vi "Dashboard Main.vi"() -> ()   [LabVIEW 2015]
uses:
  Common Code/Auton Command Cluster.ctl
  Common Code/Auton File Lists.ctl
  Vision/Camera Types.ctl
  Common Code/Goal Vision Packet.ctl
  <vilib>/Rock Robotics/WPI/Camera/WPI_CameraSettings Read MJPG.ctl
  <vilib>/Rock Robotics/WPI/Camera/WPI_CameraImageSize.ctl
  Common Code/Encoder Values Super Cluster.ctl
  Common Code/Encoder Values.ctl
  Common Code/Power and Diagnostic Data.ctl
  Common Code/Utilities/PDP Data.ctl
  Common Code/Utilities/PCM Data.ctl
  Common Code/IMU Data.ctl
  navX.Library.v2/navX Library v2/TypeDefs/Flags/Z900_navX_Flags_CalibrationStatusTypeDef.ctl
  navX.Library.v2/navX Library v2/TypeDefs/Flags/Z900_navX_Flags_OpStatusTypeDef.ctl
  Common Code/Intake Status Cluster.ctl
  Common Code/Intake Mode.ctl
  Common Code/Intake States.ctl
  Common Code/Climb Status Cluster.ctl
  Common Code/Climb Mode.ctl
  Common Code/Climb Presets.ctl
  Common Code/Major Loop Times.ctl
  Common Code/Drivetrain Settings.ctl
  Common Code/Intake Presets.ctl
  Common Code/Drivetrain Output Range.ctl
  Common Code/Ultrasonic Data.ctl
  Common Code/Autonomous Presets.ctl
  Common Code/Robot Name.ctl
  Common Code/Encoder Control.ctl
  Common Code/Drivetrain Status Cluster.ctl
  Common Code/Drivetrain Modes.ctl
  Common Code/Dist Drive Status.ctl
  Common Code/Auto Shift Cluster.ctl
  Common Code/Catapult/Catapult Presets.ctl
  Common Code/Dashboard Communication/Dashboard Control Data.ctl
  Common Code/Dashboard Drivetrain Command.ctl
  Common Code/Drivetrain Vision.ctl
  Common Code/Ball Tracking Command Cluster.ctl
  Common Code/Ball Vision Packet.ctl
  Common Code/Tracking Mode.ctl
  Common Code/IntakeEcoderControl.ctl
  Common Code/Enabled Systems.ctl
  Common Code/Dashboard Communication/Dashboard Display Data.ctl
  <vilib>/Rock Robotics/WPI/Dashboard/WPI_DashboardLogging Global.vi
  <vilib>/Utility/inputDevices.llb/keyboardAcquire.vi
  navX.Library.v2/navX Library v2/navX Library v2.lvlib
panel:
  in  "Robot":T1
  in  "Logging Filename":path=path ""
  in  "stop":bool
  out "DumbDashMessage":string="137 values loaded OK"
  in  "Save":bool
  in  "Load":bool
  in  "TCP":refnum<k5>
  in  "Rec Mode":enum32{"Stop", "Record", "Playback"}(radio)
  out "Image Message":string="Timeout in Camera Communications"
  in  "Dashboard Tab":T2(tab)
  out "Pressure":dbl
  out "Goal Active? 2":bool
  out "Drivetrain Mode":bool
  out "Intake State":bool
  out "Mode":T3(ring)=enum."Disconnected"
  out "Gyro":dbl(knob) scale=0.0..360.0 scale format="%#.7g"
  out "Climb Mode":bool
  out "Intake Mode":bool
  out "Camera IP":string="0.0.0.0"
  out "Robot IP":string="0.0.0.0"
  out "Front Camera Display":T4(plugin-control)
  in  "Camera Mode":u16(ring)=3 items=["Camera Off", "USB Camera SW", "USB Camera HW", "IP Camera"]
  out "FPS":dbl
  out "Bandwidth (Mbps)":dbl
  out "navX Calibration Status":T5 items=["IMU_CAL_STATE_MASK"=3, "IMU_CAL_STATE_INPROGRESS"=0, "IMU_CAL_STATE_ACCUMULATE"=1, "IMU_CAL_STATE_COMPLETE"=2]
  out "Front Camera Display 2":T4(plugin-control)
  out "Line Number":i32
  in  "Auton Presets":T6
  out "Auton Command Cluster":T7
  out "Auton File Lists":T8
  in  "Auto-Shift":T9
  in  "Encoder Settings":T10
  in  "Drivetrain Settings":T11={"Gyro Tolerance"=6.0, "Throttle Ramp (ms)"=250.0, "Kv"=0.0, "Ka"=0.0, "Feed Forward P"=1.0, "Feed Forward D"=0.0, "Goal Vision PID gains"={"proportional gain (Kc)"=0.8, "integral time (Ti, min)"=0.05, "derivative time (Td, min)"=0.003}, "Goal Detection Window"=12.0, "Creep Rate"=0.0, "Vision Throttle Threshold"=0.0, "Min Turn Output"=0.0, "Left Batter Angle"=0.0, "Right Batter Angle"=0.0} {"Goal Vision PID gains"."derivative time (Td, min)" format="%.5f"; "Goal Vision PID gains"."integral time (Ti, min)" format="%.3f"; "Goal Vision PID gains"."proportional gain (Kc)" format="%.3f"}
  in  "Goal Output Range":cluster{"output high":dbl, "output low":dbl}={"output high"=0.8, "output low"=-0.8}
  out "Encoder Values":T12
  in  "Steer PID output":cluster{"output high":dbl, "output low":dbl}
  in  "Steer PID gains":T14
  out "Drivetrain Status Cluster":T15={"Modes"=enum."Manual", "Y (Throttle)"=0.0, "X (Steer)"=0.0, "Gyro In Range?"=FALSE, "Distance Drive Finished?"=FALSE, "Stop Eject Lockout"=FALSE, "Dist Drive Status"={"Y In Range"=FALSE, "X In Range"=FALSE, "Gyro In Range"=FALSE, "Y Dist"=0.0, "X Dist"=0.0, "Gyro"=0.0}, "Y Target"=0.0, "Heading Target"=0.0, "Vision Target Aligned?"=FALSE}
  in  "Catapult Setpoints":T18
  in  "Intake Presets":T19={"Intake Speed"=0.8, "Outake Speed"=-0.8, "Low Height"=5.0, "Half Height"=55.0, "High Idle Height"=90.0, "Angle Speed"=0.0, "Angle Tolerance"=5.0, "Encoder Scale"=0.001478, "Load Height"=4.0, "Output Range"={"output high"=0.4, "output low"=-0.4}, "Rotation Power Max/Min"=0.5, "MaxCurrent"=40.0, "Intake Trip Time"=500.0, "Idle Height"=27.0, "Max Height"=90.0, "Reset Encoders?"=FALSE, "PID gains"={"proportional gain (Kc)"=1.0, "integral time (Ti, min)"=0.0, "derivative time (Td, min)"=0.003}, "Intake Stop Delay"=0, "Settle Time"=0.0, "Settle Wait Time"=0.0, "Pull Up Delay"=0.0} {"Pull Up Delay" format="%#_7g"; "Settle Wait Time" format="%#_7g"; "Settle Time" format="%#_7g"; "Intake Stop Delay" format="%#_7g"; "Max Height" format="%#_7g"; "Idle Height" format="%#_7g"; "Intake Trip Time" format="%#_7g"; "MaxCurrent" format="%#_7g"; "Rotation Power Max/Min" format="%#_7g"; "Load Height" format="%#_7g"; "Encoder Scale" format="%#_7g"; "Angle Tolerance" format="%#_7g"; "Angle Speed" format="%#_7g"; "High Idle Height" format="%#_7g"; "Half Height" format="%#_7g"; "Low Height" format="%#_7g"; "Outake Speed" format="%#_7g"; "Intake Speed" format="%#_7g"}
  out "Intake Status Cluster":T21
  in  "Climb Presets":T24={"Pull Power"=0.0, "Extend Power"=1.0}
  out "Climb Status Cluster":T25
  in  "Pressure B":dbl
  in  "Pressure M":dbl=22.0
  out "Pressure Sensor Voltage":dbl
  out "IMU Data":T27 {"OP Status" items=["INITIALIZING", "SELFTEST_IN_PROGRESS", "ERROR", "IMU_AUTOCAL_IN_PROGRESS", "NORMAL"]; "Calibration Status" items=["IMU_CAL_STATE_MASK"=3, "IMU_CAL_STATE_INPROGRESS"=0, "IMU_CAL_STATE_ACCUMULATE"=1, "IMU_CAL_STATE_COMPLETE"=2]}
  out "Gyro 2":dbl(knob) scale=0.0..360.0 scale format="%#.7g"
  out "Ultrasonic Data":T29
  out "Ball Cam Active?":bool
  out "Camera Display 2":T4(plugin-control)
  in  "Aspect Fudge Factor":dbl=1.0
  in  "Score Threshold 2":dbl=75.0 format="%#_13g"
  out "Goal Display":T4(plugin-control)
  out "Found Targets":T30(array[cluster]) {"Normalized Rect"."Numeric 5" format="%#_2g"; "Normalized Rect"."Numeric 3" format="%#_2g"; "Normalized Rect"."Numeric 2" format="%#_2g"; "Normalized Rect"."Numeric" format="%#_2g"}
  in  "Camera Type":T31=enum."1013"
  out "Goal Vision Packet":T32
  in  "Goal Camera Settings":T33={"fps"=30, "compression"=30, "Image Size"=enum."320x240"}
  in  "File number":i32
  in  "Use Goal File?":bool
  in  "Color Components":T35={"Hue"={34.0, 185.0}, "Sat"={0.0, 181.0}, "Val"={142.0, 255.0}} {"Val" scale=0.0..255.0; "Sat" scale=0.0..255.0; "Hue" scale=0.0..255.0 scale format="%#_3g"}
  out "Goal Active?":bool
  in  "Camera Mode 2":u16(ring) items=["Camera Off", "USB Camera SW", "USB Camera HW", "IP Camera"]
  out "FPS 2":dbl
  out "Bandwidth (Mbps) 2":dbl
  in  "Ball Camera Settings":T33={"fps"=30, "compression"=30, "Image Size"=enum."320x240"}
  out "Front Camera Display 3":T4(plugin-control)
  in  "Vision Timeout":dbl
  out "Power and Diagnostic Data":T36
  out "Control Info":T39
  out "Status Info":T40
  out "DS TCP":T41={"Error Strings"="", "Disable Counts"={0, 0}, "Rail Faults"={0, 0, 0}, "Robot IP"="0.0.0.0", "DB Mode"=4, "Event Info"={"Name"="", "Type"=0, "Number"=0, "Replay"=0}, "Camera Addr"="0.0.0.0"}
  out "Robot Metrics":T42
  out "Loop Times":T43
  # "USB Cam"
  # "Axis Cam"
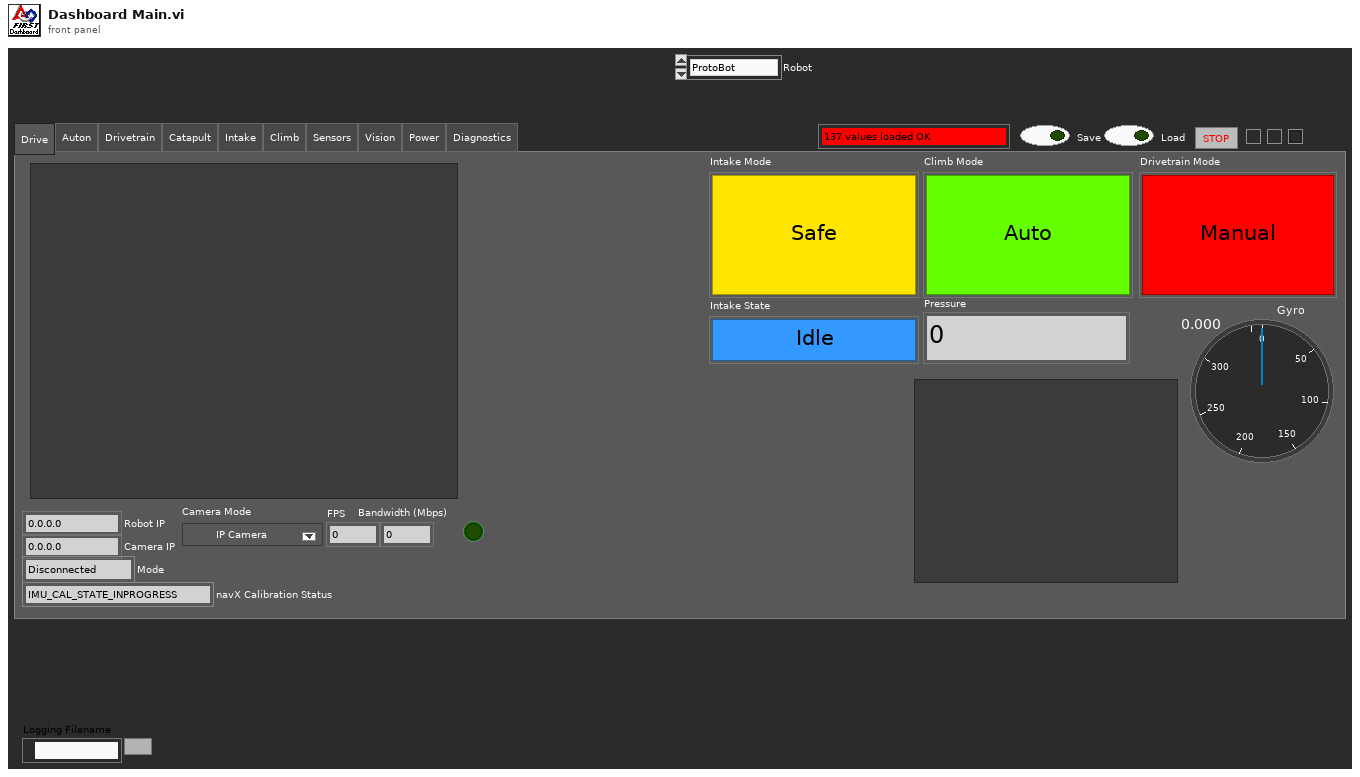
[diagram p1: front panel]
types:
  T1 = typedef "Robot Name.ctl" = enum16{"ProtoBot", "Main Robot", "Practice Robot"}
  T2 = enum32{"Drive", "Auton", "Drivetrain", "Catapult", "Intake", "Climb", "Sensors", "Vision", "Power", "Diagnostics"}
  T3 = enum8{"Tele-Op Disabled", "Tele-Op Enabled", "Auto Disabled", "Auto Enabled", "Test Disabled", "Test Enabled", "Disconnected", "No Code", "E-Stop"}
  T4 = typedef "IMAQ Image.ctl" = refnum<image>
  T5 = typedef "navX Library v2.lvlib/Z900_navX_Flags_CalibrationStatusTypeDef.ctl" = u8
  T6 = typedef "Autonomous Presets.ctl" = cluster{"Pitch Limit":dbl, "Roll Limit":dbl, "Start Position":dbl, "Cross Position":dbl}
  T7 = typedef "Auton Command Cluster.ctl" = cluster{"Command ID":i32, "maxTime":dbl, "Y Distance":dbl, "Heading":dbl, "Throttle":dbl, "Async":dbl, "Velocity":dbl, "Acceleration":dbl, "To":dbl, "Condition":dbl, "Shot Type":dbl, "Left RPM":dbl, "Override RPM":i32, "Override Angle":i32, "Right RPM":dbl, "Angle":dbl, "Intake Mode":i32, "Intake Cmd":i32, "Intake O":i32, "Eject O":i32, "Angle O":i32, "Arm O":i32, "Intake Speed":dbl, "Eject Speed":dbl, "Arm Angle":dbl, "Arm Speed":dbl, "Intake?":i32, "Eject?":i32, "Left":dbl, "Right":dbl, "Pivot Speed":dbl, "Y Dist":dbl, "Position":dbl, "Desired Position":i32, "Shooter Mode":dbl, "Shooter Command":dbl, "Shoot?":dbl, "Shoot mode":dbl}
  T8 = typedef "Auton File Lists.ctl" = cluster{"Current Queue":string, "General Scripts":string, "Defense Scripts":string, "Movement Scripts":string}
  T9 = typedef "Auto Shift Cluster.ctl" = cluster{"Delay":dbl, "Speed Thresh":dbl, "Upshift Accel":dbl, "Upshift Throttle":dbl, "Upshift Throttle Accel":dbl, "Downshift Throttle":dbl, "Downshift Throttle Accel":dbl, "Pressure Threshold":dbl}
  T10 = typedef "Encoder Control.ctl" = cluster{"Right Tick Constant":dbl, "Left Tick Constant":dbl, "Reset?":bool, "Y Dist":cluster{"PID gains":cluster{"proportional gain (Kc)":dbl, "integral time (Ti, min)":dbl, "derivative time (Td, min)":dbl}}, "Y Stop Thresh":dbl, "Y Stop Speed":dbl}
  T11 = typedef "Drivetrain Settings.ctl" = cluster{"Gyro Tolerance":dbl, "Throttle Ramp (ms)":dbl, "Kv":dbl, "Ka":dbl, "Feed Forward P":dbl, "Feed Forward D":dbl, "Goal Vision PID gains":cluster{"proportional gain (Kc)":dbl, "integral time (Ti, min)":dbl, "derivative time (Td, min)":dbl}, "Goal Detection Window":dbl, "Creep Rate":dbl, "Vision Throttle Threshold":dbl, "Min Turn Output":dbl, "Left Batter Angle":dbl, "Right Batter Angle":dbl}
  T12 = typedef "Encoder Values Super Cluster.ctl" = cluster{"Left Encoder":T13, "Right Encoder":T13}
  T13 = typedef "Encoder Values.ctl" = cluster{"Distance":dbl, "Speed":dbl, "Ticks":dbl}
  T14 = cluster{"proportional gain (Kc)":dbl, "integral time (Ti, min)":dbl, "derivative time (Td, min)":dbl}
  T15 = typedef "Drivetrain Status Cluster.ctl" = cluster{"Modes":T16, "Y (Throttle)":dbl, "X (Steer)":dbl, "Gyro In Range?":bool, "Distance Drive Finished?":bool, "Stop Eject Lockout":bool, "Dist Drive Status":T17, "Y Target":dbl, "Heading Target":dbl, "Vision Target Aligned?":bool}
  T16 = typedef "Drivetrain Modes.ctl" = enum16{"Gyro Steer", "Climb", "Manual", "Goal Vision Targeting", "PID Distance Drive", "Hybrid"}
  T17 = typedef "Dist Drive Status.ctl" = cluster{"Y In Range":bool, "X In Range":bool, "Gyro In Range":bool, "Y Dist":dbl, "X Dist":dbl, "Gyro":dbl}
  T18 = typedef "Catapult Presets.ctl" = cluster{"Intake Danger Height":dbl, "Ball Security Delay ":dbl, "High PSI Minimum":dbl, "Shot Finish Delay":dbl, "Low PSI Minimum":dbl, "Idle Ball Security Wait ":dbl}
  T19 = typedef "Intake Presets.ctl" = cluster{"Intake Speed":dbl, "Outake Speed":dbl, "Low Height":dbl, "Half Height":dbl, "High Idle Height":dbl, "Angle Speed":dbl, "Angle Tolerance":dbl, "Encoder Scale":dbl, "Load Height":dbl, "Output Range":T20, "Rotation Power Max/Min":dbl, "MaxCurrent":dbl, "Intake Trip Time":dbl, "Idle Height":dbl, "Max Height":dbl, "Reset Encoders?":bool, "PID gains":cluster{"proportional gain (Kc)":dbl, "integral time (Ti, min)":dbl, "derivative time (Td, min)":dbl}, "Intake Stop Delay":u32, "Settle Time":dbl, "Settle Wait Time":dbl, "Pull Up Delay":dbl}
  T20 = typedef "Drivetrain Output Range.ctl" = cluster{"output high":dbl, "output low":dbl}
  T21 = typedef "Intake Status Cluster.ctl" = cluster{"Roller Power":dbl, "Angle Power":dbl, "Intake Mode":T22, "Intake States":T23, "Rollers Active?":bool, "Current Height":dbl, "Target Height":dbl, "Encoder Raw Position":dbl, "Forward Tripped?":bool, "Backward Tripped?":bool, "Override IR?":bool}
  T22 = typedef "Intake Mode.ctl" = enum16{"Safe", "Auto", "Manual"}
  T23 = typedef "Intake States.ctl" = enum16{"Idle", "Set roller speed", "Move to angle", "Go Hard or Go Home", "Ball Settle"}
  T24 = typedef "Climb Presets.ctl" = cluster{"Pull Power":dbl, "Extend Power":dbl}
  T25 = typedef "Climb Status Cluster.ctl" = cluster{"Pull Power":dbl, "Unpin Power":dbl, "PTO Engaged?":bool, "Climb Mode":T26}
  T26 = typedef "Climb Mode.ctl" = enum16{"Auto", "Semi-Auto", "Manual"}
  T27 = typedef "IMU Data.ctl" = cluster{"Pitch":sgl, "Roll":sgl, "Yaw":sgl, "Data Valid?":bool, "Temp":sgl, "MOVING":bool, "YAW_STABLE":bool, "Accel X":sgl, "Accel Y":sgl, "Accel Z":sgl, "Accel Magnitude":sgl, "Pitch Rate":sgl, "Roll Rate":sgl, "Yaw Rate":sgl, "NavX Opened?":bool, "Calibration Status":T5, "OP Status":T28}
  T28 = typedef "navX Library v2.lvlib/Z900_navX_Flags_OpStatusTypeDef.ctl" = u8
  T29 = typedef "Ultrasonic Data.ctl" = cluster{"Left Ultrasonic":dbl, "Right Ultrasonic":dbl}
  T30 = cluster{"Distance (ft)":dbl, "Center":cluster{dbl, dbl}, "Normalized Rect":cluster{"Numeric":dbl, "Numeric 2":dbl, "Numeric 3":dbl, "Numeric 5":dbl}}[]
  T31 = typedef "Camera Types.ctl" = enum16{"206", "1011", "1013", "MS HD3000 square", "MS HD3000 640x480"}
  T32 = typedef "Goal Vision Packet.ctl" = cluster{"Distance":dbl, "Center X":dbl, "Center Y":dbl, "Found Target?":bool, "Robot Center":dbl, "Angle":dbl}
  T33 = typedef "WPI_CameraSettings Read MJPG.ctl" = cluster{"fps":i32, "compression":i32, "Image Size":T34}
  T34 = typedef "WPI_CameraImageSize.ctl" = enum16{"640x480", "320x240", "160x120", "Custom"}
  T35 = cluster{"Hue":cluster{dbl, dbl}, "Sat":cluster{dbl, dbl}, "Val":cluster{dbl, dbl}}
  T36 = typedef "Power and Diagnostic Data.ctl" = cluster{"PDP Data":T37, "PCM Data":T38, "roboRIO input voltage (V)":dbl, "roboRIO input current (A)":dbl, "3.3V Rail Short":bool, "5 V Rail Short":bool, "6 V Rail Short":bool, "roboRIO Brownout":bool, "Outputs Enabled?":bool}
  T37 = typedef "PDP Data.ctl" = cluster{"Battery Voltage":sgl, "Temperature (degrees C)":sgl, "Internal Battery R (Ohms)":sgl, "Energy (J)":sgl, "Power (W)":sgl, "Total Current (A)":sgl, "Battery Voltage Fault":bool, "Temperature Fault":bool, "Hardware Fault":bool, "Currents":cluster{"[0]":sgl, "[1]":sgl, "[2]":sgl, "[3]":sgl, "[4]":sgl, "[5]":sgl, "[6]":sgl, "[7]":sgl, "[8]":sgl, "[9]":sgl, "[10]":sgl, "[11]":sgl, "[12]":sgl, "[13]":sgl, "[14]":sgl, "[15]":sgl}, "Current Faults":cluster{"[0]":bool, "[1]":bool, "[2]":bool, "[3]":bool, "[4]":bool, "[5]":bool, "[6]":bool, "[7]":bool, "[8]":bool, "[9]":bool, "[10]":bool, "[11]":bool, "[12]":bool, "[13]":bool, "[14]":bool, "[15]":bool}}
  T38 = typedef "PCM Data.ctl" = cluster{"Compressor Fault":bool, "Solenoid Fault":bool, "Compressor Enabled":bool, "Hardware Fault":bool, "Compressor Current":dbl}
  T39 = cluster{"Control Bits":cluster{"TestMode":bool, "Autonomous":bool, "Enabled":bool, "FMS Present":bool, bool, bool, bool, "E-Stop":bool}, "Team Station ":u8, "Countdown":sgl, "Joystick Values":cluster{"Axes":dbl[], "Buttons":bool[], "POVs":i16[]}[]}
  T40 = cluster{"Status bits":cluster{"Test Mode":bool, "Autonomous":bool, "Enabled":bool, "Code Start":bool, "Brownout":bool, "Reserved 2":bool, "Reserved 3":bool, "E-Stop":bool}, "Code Trace":cluster{"Disabled":bool, "TeleOp":bool, "Auto":bool, "Test":bool}, "Controller Type":enum16{"unknown", "cRIO", "roboRio"}, "Code?":enum16{"unknown", "noCode", "code"}, "Battery V":dbl}
  T41 = cluster{"Error Strings":string, "Disable Counts":cluster{u16, u16}, "Rail Faults":cluster{u16, u16, u16}, "Robot IP":string, "DB Mode":u8, "Event Info":cluster{"Name":string, "Type":u8, "Number":u16, "Replay":u8}, "Camera Addr":string}
  T42 = cluster{"Storage":cluster{"Disk Free":u64, "RAM Block":u32, "RAM free":u32}, "CPU Utilization":cluster{"CPU % ISR":sgl, "CPU % Time Crit":sgl, "CPU % Timed Str":sgl, "CPU % High":sgl, "CPU % Above":sgl, "CPU % Normal":sgl, "CPU % Low":sgl}, "CAN":cluster{"% Bus Utilization":sgl, "Bus Off Cnt":u32, "TX_FIFO Full Cnt":u32, "Receive Error Cnt":u8, "Transmit Error Cnt":u8}, "HID":cluster{"HID Outputs":u32, "Rumble Low":u16, "Rumble High":u16}[]}
  T43 = typedef "Major Loop Times.ctl" = cluster{"DT Loop Timer":u32, "Shooter Loop Timer":u32, "Intake Loop Timer":u32, "US Loop Timer":u32, "Auton File Loop Timer":u32}
  T44 = typedef "Image Type" = u32
  T45 = typedef "NI_LVConfig.lvlib/Config Data RefNum.ctl" = refnum<k1>
  T46 = cluster{cluster{dbl, dbl}, cluster{dbl, dbl}, cluster{dbl, dbl}}
  T47 = cluster{"Bounding box":cluster{"left":dbl, "top":dbl, "right":dbl, "bottom":dbl}, "Aspect Ratio":dbl, "Area to CH":dbl, "X Mask":dbl, "Y Mask":dbl, "Moment":dbl}[]
  T48 = cluster{"Distance (ft)":dbl, "Center":cluster{dbl, dbl}, "Normalized Rect":cluster{"Numeric":dbl, "Numeric 2":dbl, "Numeric 3":dbl, "Numeric 5":dbl}}
  T49 = typedef "Dashboard Display Data.ctl" = cluster{"Auton Command Cluster":T7, "Auton File Lists":T8, "Drivetrain Status Cluster":T15, "Encoder Values":T12, "IMU Data":T27, "Power and Diagnostic Data":T36, "Gyro":dbl, "Intake Status Cluster":T21, "Ultrasonic Data":T29, "Climb Status Cluster":T25, "Loop Times":T43, "Pressure":dbl, "Pressure Voltage":dbl, "Auton Line Number":i32}
  T50 = typedef "Dashboard Control Data.ctl" = cluster{"Encoder Control":T10, "Steer PID output":cluster{"output high":dbl, "output low":dbl}, " Steer PID gains":cluster{"proportional gain (Kc)":dbl, "integral time (Ti, min)":dbl, "derivative time (Td, min)":dbl}, "Drivetrain Settings":T11, "Vision Packet":T32, "Dashboard Drivetrain Command":T51, "Info/Command Cluster":T53, "Ball Vision Packet":T54, "Intake Presets":T19, "Intake Encoder Control":T56, "Climb Presets":T24, "Goal Output Range":cluster{"output high":dbl, "output low":dbl}, "Enabled Systems":T57, "Auton Presets":T6, "Pressure M":dbl, "Pressure B":dbl, "Vision Timeout":dbl, "Auto-Shift":T9, "Catapult Setpoints":T18}
  T51 = typedef "Dashboard Drivetrain Command.ctl" = cluster{"Drivetrain Vision":T52}
  T52 = typedef "Drivetrain Vision.ctl" = cluster{"Goal Window":dbl, "Ball Window":dbl}
  T53 = typedef "Ball Tracking Command Cluster.ctl" = cluster{"Distance to Ball":dbl, "Desired Angle":dbl, "Command":enum16{"Turn to Ball", "Turn to Angle", "Get Distance"}, "Pixels from Center":dbl}
  T54 = typedef "Ball Vision Packet.ctl" = cluster{"Ball Detected?":bool, "Distance to Ball":dbl, "Desired Angle":dbl, "Pixels from Center":dbl, "Tracking mode":T55}
  T55 = typedef "Tracking Mode.ctl" = enum16{"Turn to Ball", "Turn to Angle"}
  T56 = typedef "IntakeEcoderControl.ctl" = cluster{"Arm Tick Constant":dbl, "Reset?":bool, "Y Dist":cluster{"PID gains":cluster{"proportional gain (Kc)":dbl, "integral time (Ti, min)":dbl, "derivative time (Td, min)":dbl}}, "Y Stop Thresh":dbl, "Y Stop Speed":dbl}
  T57 = typedef "Enabled Systems.ctl" = cluster{"Shoot":bool, "Intake":bool, "DT":bool, "Gyro":bool, "100ms":bool, "US":bool}
  T58 = cluster{"Image Size":bool, "Image Type":bool, "Pixel Value":bool, "ROI Information":bool, "Zoom Factor":bool}
  T59 = enum16{"0", "1", "2", "3", "4", "5", "6", "7", "8", "9", "A", "B", "C", "D", "E", "F", "G", "H", "I", "J", "K", "L", "M", "N", "O", "P", "Q", "R", "S", "T", "U", "V", "W", "X", "Y", "Z", "F1", "F2", "F3", "F4", "F5", "F6", "F7", "F8", "F9", "F10", "F11", "F12", "F13", "F14", "F15", "ADD", "BACK", "BACKSLASH", "CAPITAL", "COMMA", "DECIMAL", "DELETE", "DIVIDE", "DOWN", "END", "EQUALS", "ESCAPE", "GRAVE (`)", "HOME", "INSERT", "LBRACKET", "LCONTROL", "LEFT", "L ALT", "LSHIFT", "LWIN", "MINUS", "MULTIPLY", "NEXT", "NUMLOCK", "NUMPAD_0", "NUMPAD_1", "NUMPAD_2", "NUMPAD_3", "NUMPAD_4", "NUMPAD_5", "NUMPAD_6", "NUMPAD_7", "NUMPAD_8", "NUMPAD_9", "PAUSE", "PERIOD", "PRIOR (PG UP)", "RBRACKET", "RCONTROL", "RETURN", "RIGHT", "R ALT", "RSHIFT", "RWIN", "SCROLL", "SEMICOLON", "SLASH", "SPACE", "SUBTRACT", "TAB", "UP", "ENTER (num pad)", "' (quote)"}[]
  T60 = typedef "DumbDash Control.ctl" = cluster{"Name":string, "Ref":refnum<vi>, "Type":T61}
  T61 = typedef "DumbDash Control Type.ctl" = enum16{"Invalid", "Number", "Boolean", "String"}
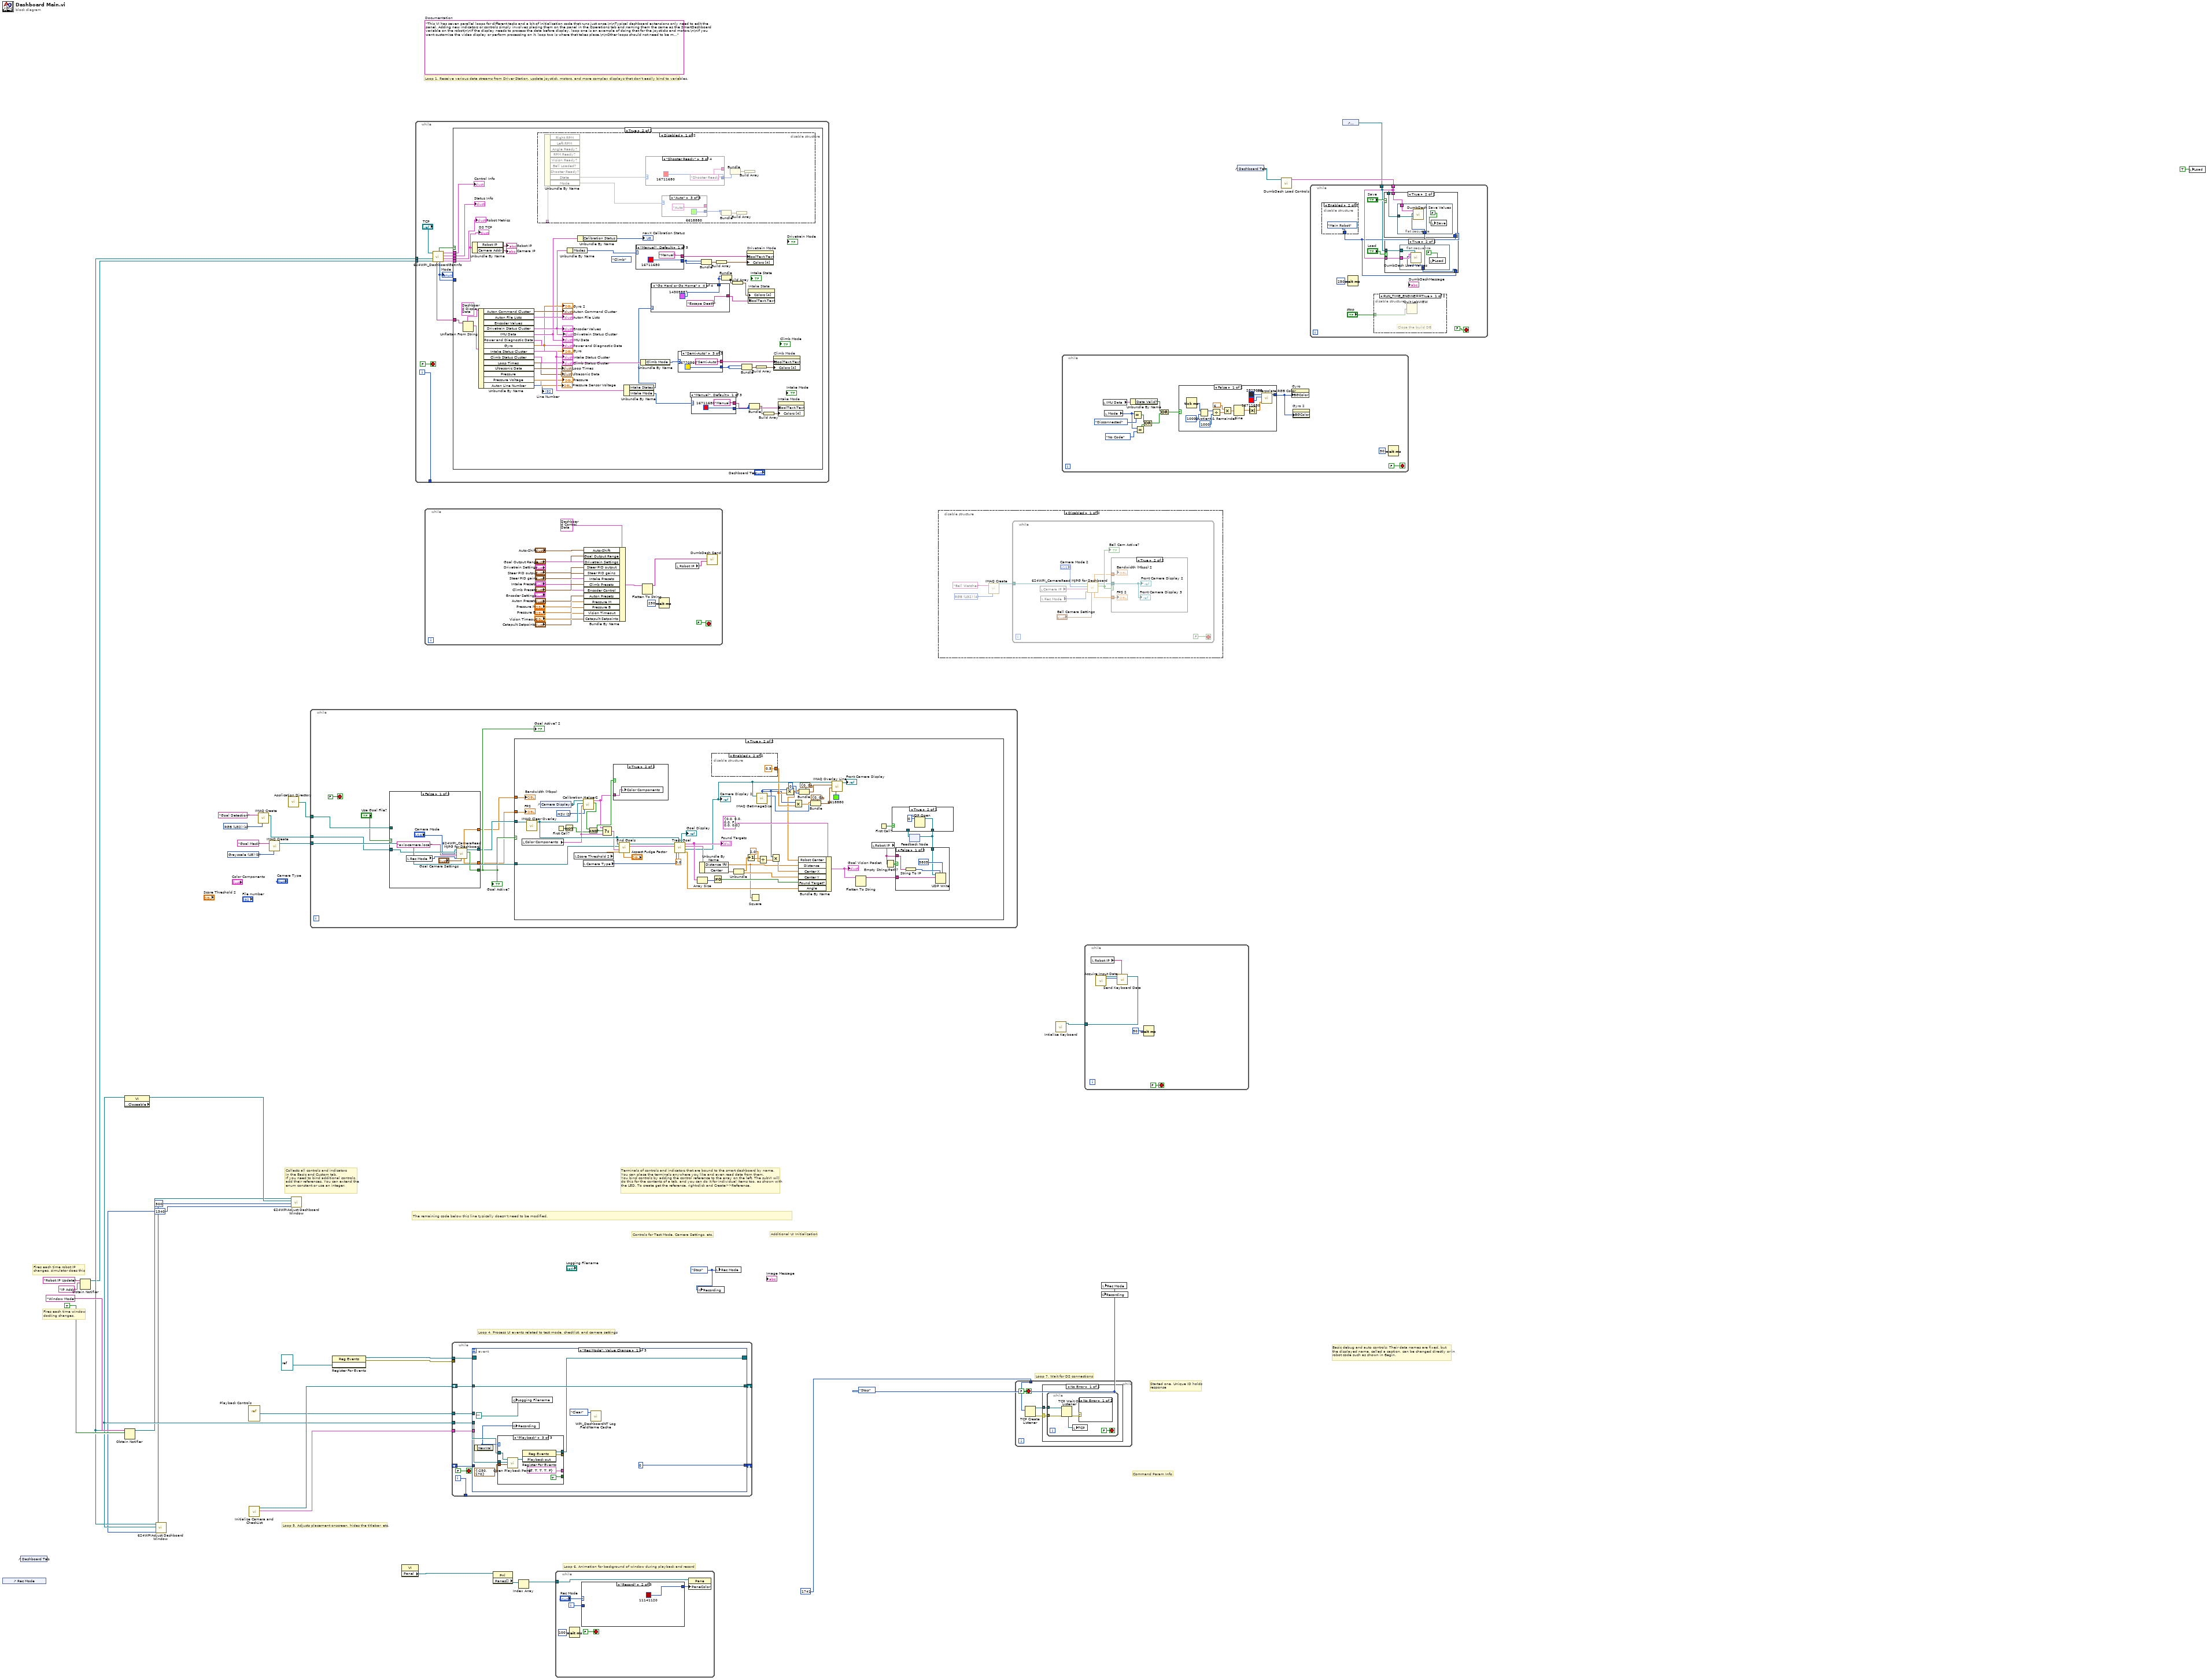
[diagram p0: block diagram]
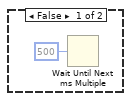
[diagram p2: hidden frame]
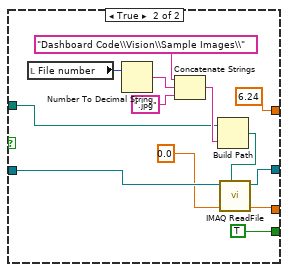
[diagram p4: hidden frame]
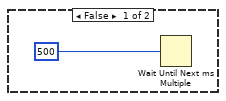
[diagram p5: hidden frame]
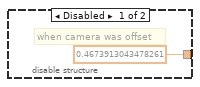
[diagram p9: hidden frame]
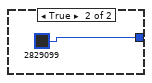
[diagram p10: hidden frame]
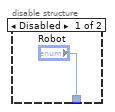
[diagram p11: hidden frame]
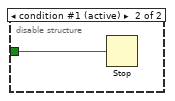
[diagram p12: hidden frame]
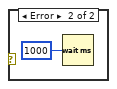
[diagram p15: hidden frame]
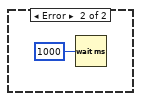
[diagram p16: hidden frame]
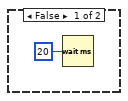
[diagram p17: hidden frame]
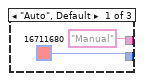
[diagram p18: hidden frame]
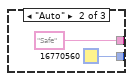
[diagram p19: hidden frame]
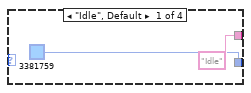
[diagram p20: hidden frame]
diagram:
  w3 = T44 0 items=["Grayscale (U8)", "Grayscale (I16)", "Grayscale (SGL)", "Complex (CSG)", "RGB (U32)", "HSL (U32)", "RGB (U64)", "Grayscale (U16)"] ("Image Type")
  w7 = T44 4 items=["Grayscale (U8)", "Grayscale (I16)", "Grayscale (SGL)", "Complex (CSG)", "RGB (U32)", "HSL (U32)", "RGB (U64)", "Grayscale (U16)"] ("Image Type")
  w10 = enum16{"Stop", "Record", "Playback"}."Stop"
  w15 = 1340
  w16 = 500
  w20 = enum32{"Stop", "Record", "Playback"}."Stop" ("Rec Mode")
  (unwired) "This VI has seven parallel loops for different tasks and a bit of initialization code that runs just once.\n\nTypical dashboard extensions only need to edit the panel. Adding new indicators or controls simply involves placing them on the panel in the Operations tab and naming them the same as the SmartDashboard variable on the robot\n\nIf the display needs to process the data before display, loop one is an example of doing that for the joysticks and motors.\n\nIf you want customize the video display or perform processing on it, loop two is where that takes place.\n\nOther loops should not need to be modified. They are pretty standard, and document the task they perform."  # Documentation
  # "Command Param Info"
  # "Started one, Unique ID holds\nresponse"
  # "Loop 7. Wait for DS connections"
  # "Basic debug and auto controls: Their data names are fixed, but\nthe displayed name, called a caption, can be changed directly or in\nrobot code such as shown in Begin."
  # "Controls for Test Mode, Camera Settings, etc."
  # "Additional UI Initialization"
  # "Loop 6. Animation for background of window during playback and record"
  # "Fires each time robot IP\nchanges, simulator does this"
  # "Fires each time window\ndocking changes."
  # "Collects all controls and indicators\nin the Basic and Custom tab.\nIf you need to bind additional controls,\nadd their references. You can extend the\nenum constant or use an integer."
  # "The remaining code below this line typically doesn't need to be modified."
  # "Loop 4. Process UI events related to test mode, checklist, and camera settings"
  # "Terminals of controls and indicators that are bound to the smart dashboard by name.\nYou can place the terminals anywhere you like and even read data from them.\nYou bind controls by adding the control reference to the array on the left. The subVI will\ndo this for the contents of a tab, and you can do it for individual items too, as shown with\nthe LED. To create get the reference, right-click and Create>>Reference."
  # "Loop 5. Adjusts placement onscreen, hides the titlebar, etc."
  # "Loop 1. Receive various data streams from Driver Station, update joystick, motors, and more complex displays that don't easily bind to variables."
  n1 = control-ref of="Rec Mode"() -> ()  [unwired: 1 out]
  n2 = control-ref of="Dashboard Tab"() -> ()  [unwired: 1 out]
  n3 = Obtain Notifier(name (unnamed)="Robot IP Update", notification data type="IP Addr" ("name (unnamed)")) -> (notifier out=w14:refnum<notifier>)  [unwired: 2 in, 2 out]
  n4 = property class="VI" props=["Front Panel.Closeable"]() -> (reference out=w19:refnum<vi>)  [unwired: 2 in, 2 out]
  n5 = Obtain Notifier(name (unnamed)="Window Mode", notification data type=TRUE) -> (notifier out=w18:refnum<notifier>)  [unwired: 2 in, 2 out]
  n6 = call "624WPIAdjust Dashboard Window.vi"("Width"=w15, "Height"=w16, "VI"=w19, "Notifier in"=w18) -> ()  [unwired: 8 in]
  n7 = vi-ref "Playback Controls.vi"() -> (w24:refnum<vi>)
  n8 = call "Initialize Camera and CheckList.vi"() -> ("Array"=w29:cluster{string[]}[], "File Refnum"=w28:T45)  [unwired: 9 in, 1 out]
  n9 = call "IMAQ Create"("Image Name"="Goal Detection", "Image Type"=w7) -> ("New Image"=w8:T4)  [unwired: 3 in, 1 out]
  n10 = call "IMAQ Create"("Image Name"="Goal Mask", "Image Type"=w3) -> ("New Image"=w5:T4)  [unwired: 3 in, 1 out]
  n11 = call <vilib>:"Application Directory.vi"() -> ("Application Directory"=w2:path)
  n12 = call "624WPIAdjust Dashboard Window.vi"("Width"=w15, "Height"=w16, "VI"=w19, "Notifier in"=w18) -> ()  [unwired: 8 in]
  n13 = while {
    tunnel: w5 -> [w42]
    tunnel: w8 -> [w40]
    tunnel: w2 -> [w38]
    stop <- FALSE stop-if-true
    n14 = case shown="False" "Use Goal File?" {
      tunnel: [w46 TRUE] -> w41
      tunnel: w40 -> [w51 w62]
      tunnel: [w45 w61] -> w39
      tunnel: w38 -> [_ w56]
      tunnel: [w43 6.24 ("Bandwidth (Mbps)")] -> w36
      tunnel: [w44 0.0 ("FPS")] -> w35
      frame False {
        n15 = local read "Rec Mode"() -> (w48:enum32{"Stop", "Record", "Playback"})
        n16 = call "624WPI_CameraRead MJPG for Dashboard.vi"("Camera Settings"="Goal Camera Settings", "Rec Mode"=w48, "Camera IP"="axis-camera.local", "Camera Mode"="Camera Mode", "Refnum in"=w51) -> ("Active"=w46:bool, "Refnum out"=w45:T4, "FPS"=w44:dbl, "Bandwidth (Mbps)"=w43:dbl)  [unwired: 3 in]
      }
      frame True {
        n17 = local read "File number"() -> (w54:i32)
        n18 = Number To Decimal String(number=w54) -> (decimal integer string=w59:string)  [unwired: 1 in]
        n19 = Concatenate Strings("Dashboard Code\\Vision\\Sample Images\\", w59, ".jpg" ("string")) -> (w57:string)
        n20 = Build Path(base path=w56, name or relative path=w57) -> (appended path=w55:path)
        n21 = call "IMAQ ReadFile"("File Path"=w55, "Image"=w62) -> ("Image Out"=w61:T4)  [unwired: 5 in, 4 out]
      }
    }
    "Goal Active?" <- w41
    "Goal Active? 2" <- w41
    n22 = case shown="True" w41 {
      tunnel: w39 -> [_ w118]
      tunnel: w42 -> [_ w99]
      tunnel: w36 -> [_ w107]
      tunnel: w35 -> [_ w106]
      frame False {
        n23 = Wait Until Next ms Multiple(millisecond multiple=u32 500) -> ()  [unwired: 1 out]
      }
      frame True {
        w102 = u16 2 items=["RGB", "HSL", "HSV", "HSI", "CIE L*a*b*", "CIE XYZ"] ("Color Mode")
        n24 = local read "Color Components"() -> (w103:T35)
        n25 = call "IMAQ Clear Overlay"("Image"=w118) -> ("Image Out"=w105:T4)  [unwired: 9 in, 1 out]
        n26 = control-ref of="Camera Display 2"() -> (w104:refnum<vi>)
        n27 = First Call?() -> (First Call?: T/F=w69:bool)
        n28 = Not(x=w69) -> (.not. x?=w68:bool)
        n29 = local read "Score Threshold 2"() -> (w119:dbl)
        n30 = call "Calibration Helper2.vi"("Color Mode"=w102, "Color Components"=w103, "Image"=w105, "Image Ctl Refnum"=w104) -> ("Changed"=w67:bool, "output color"=w65:T46)  [unwired: 6 in]
        n31 = local read "Camera Type"() -> (w115:T31)
        n32 = And(x=w67, y=w68) -> (x .and. y?=w66:bool)
        n33 = Select(t=w65, s=w66, f=w103) -> (s? t:f=w101:T35)
        n34 = case shown="True" w66 {
          tunnel: w65 -> [_ w120]
          frame False {
          }
          frame True {
            n35 = local write "Color Components"(w120) -> ()
          }
        }
        n36 = call "Find Goals.vi"("Aspect Fudge Factor"="Aspect Fudge Factor", "Score Threshold"=w119, "Color"=w101, "Image Dst"=w99, "Image Src"=w105) -> ("Targets"=w117:T47, "Masked Image"=w116:T4)  [unwired: 5 in]
        n37 = call "Track Goal.vi"("Offset"=0.0, "Original Image"=w105, "Camera Type"=w115, "Targets"=w117, "Goal Display"=w116) -> ("Angle Difference"=w81:dbl, "Target Line Masking Out"=w90:T4, "Best Target Available"=w114:T48, "Found Targets"=w109:T30, "Goal Display"=→"Goal Display":T4)  [unwired: 2 in]
        "Found Targets" <- w109
        "Camera Display 2" <- w90
        n38 = Array Size(array=w109) -> (size(s)=w110:i32)
        n39 = Unbundle By Name(w114) -> ("Distance (ft)"=w78:dbl, "Center"=w112:cluster{dbl, dbl})
        n40 = disable-structure shown="Enabled" {
          disable-tunnel: [0.4673913043478261 0.5] -> w89
          frame Disabled {
            # "when camera was offset"
          }
          frame Enabled {
          }
        }
        n41 = Not Equal To 0?(x=w110) -> (x != 0?=w108:bool)
        n42 = Unbundle(w112) -> (w88:dbl, w111:dbl)
        n43 = Increment(x=w88) -> (x+1=w87:dbl)
        n44 = Square(x=w78) -> ()  [unwired: 1 out]
        n45 = call "IMAQ GetImageSize"("Image"=w90) -> ("Y Resolution"=w92:i32, "X Resolution"=w83:i32)  [unwired: 3 in, 1 out]
        n46 = Divide(x=w87, y=2.0) -> (x/y=w85:dbl)
        n47 = Multiply(x=w83, y=w85) -> (x*y=w84:dbl)
        n48 = Multiply(x=w83, y=w89) -> (x*y=w82:dbl)
        n49 = Multiply(x=w83, y=w89) -> (x*y=w95:dbl)
        n50 = Bundle By Name(cluster=T32 {"Distance"=0.0, "Center X"=0.0, "Center Y"=0.0, "Found Target?"=FALSE, "Robot Center"=0.0, "Angle"=0.0}, "Robot Center"=w82, "Distance"=w78, "Center X"=w84, "Center Y"=w111, "Found Target?"=w108, "Angle"=w81) -> (w71:T32)
        "Goal Vision Packet" <- w71
        n51 = Bundle(cluster=cluster{"X":i32, "Y":i32} {"X"=0, "Y"=0} ("Start Point"), "X"=w82, "Y"=0) -> (w94:cluster{"X":i32, "Y":i32})
        n52 = Bundle(cluster=cluster{"X":i32, "Y":i32} {"X"=0, "Y"=0} ("Start Point"), "X"=w95, "Y"=w92) -> (w93:cluster{"X":i32, "Y":i32})
        n53 = call "IMAQ Overlay Line"("Color"=u32 6618880, "End Point"=w93, "Start Point"=w94, "Image"=w90) -> ("Image Out"=→"Front Camera Display":T4)  [unwired: 6 in, 1 out]
        n54 = Flatten To String(anything=w71) -> (data string=w70:string)  [unwired: 3 in, 2 out]
        n55 = local read "Robot IP"() -> (w72:string)
        n56 = First Call?() -> (First Call?: T/F=w75:bool)
        n57 = Empty String/Path?(string/path=w72) -> (empty?=w76:bool)
        n58 = feedback #1() -> (w73:refnum<k16>)  [unwired: 1 in]
        n59 = case shown="True" w75 {
          tunnel: [w121 w123] -> w74
          tunnel: w73 -> [w121 _]
          frame False {
          }
          frame True {
            n60 = UDP Open(11:u16 0 ("port")) -> (port=w123:refnum<k16>)  [unwired: 4 in, 2 out]
          }
        }
        n61 = case shown="False" w76 {
          tunnel: w72 -> [w126 _]
          tunnel: w70 -> [w125 _]
          tunnel: w74 -> [w124 _]
          frame False {
            n62 = String To IP(1:w126) -> (0:w127:u32)
            n63 = UDP Write(address=w127, port or service name=u16 5805, connection ID=w124, data in=w125) -> ()  [unwired: 2 in, 2 out]
          }
          frame True {
            # "The robot IP is not\nready yet, don't try\nto send data"
          }
        }
        n64 = feedback-in #1(w74) -> ()
        "Bandwidth (Mbps)" <- w107
        "FPS" <- w106
      }
    }
  }
  n65 = register-events(refnum<vi> refnum) -> (reference out=w23:refnum<event-registration>, error out=w22:errorcluster)  [unwired: 2 in]
  n66 = property class="VI"() -> ("Panel"=w26:refnum<vi>)  [unwired: 2 in, 2 out]
  n67 = while {
    tunnel: [w141] -> _
    tunnel: w14 -> [w140]
    tunnel: w18 -> [w138]
    i -> [w141]
    stop <- FALSE stop-if-true
    n68 = call "624WPI_DashboardGetInfo.vi"("Binding Refnum"=w140, "Window Mode Notifier"=w138, "TCP Cnx"="TCP") -> ("Power and Errors"=w137:T41, "Robot Metrics"=w136:T42, "Status Info"=w135:T40, "Control Info"=w134:T39, "Robot Mode"=w133:T3, "Process?"=w132:bool, "Custom Dashboard Data"=w131:string)  [unwired: 2 in]
    "Mode" <- w133
    n69 = case shown="True" w132 {
      tunnel: w135 -> [_ w186]
      tunnel: w136 -> [_ w185]
      tunnel: w134 -> [_ w187]
      tunnel: w137 -> [_ w184]
      tunnel: w133 -> [_ _]
      tunnel: w131 -> [_ w181]
      frame False {
        n70 = Wait (ms)(milliseconds to wait=u32 20) -> ()  [unwired: 1 out]
      }
      frame True {
        (unwired) Drivetrain_Modes."Climb" ("Modes")
        n71 = Unflatten From String(type=T49 {"Auton Command Cluster"={"Command ID"=0, "maxTime"=0.0, "Y Distance"=0.0, "Heading"=0.0, "Throttle"=0.0, "Async"=0.0, "Velocity"=0.0, "Acceleration"=0.0, "To"=0.0, "Condition"=0.0, "Shot Type"=0.0, "Left RPM"=0.0, "Override RPM"=0, "Override Angle"=0, "Right RPM"=0.0, "Angle"=0.0, "Intake Mode"=0, "Intake Cmd"=0, "Intake O"=0, "Eject O"=0, "Angle O"=0, "Arm O"=0, "Intake Speed"=0.0, "Eject Speed"=0.0, "Arm Angle"=0.0, "Arm Speed"=0.0, "Intake?"=0, "Eject?"=0, "Left"=0.0, "Right"=0.0, "Pivot Speed"=0.0, "Y Dist"=0.0, "Position"=0.0, "Desired Position"=0, "Shooter Mode"=0.0, "Shooter Command"=0.0, "Shoot?"=0.0, "Shoot mode"=0.0}, "Auton File Lists"={"Current Queue"="", "General Scripts"="", "Defense Scripts"="", "Movement Scripts"=""}, "Drivetrain Status Cluster"={"Modes"=enum."Manual", "Y (Throttle)"=0.0, "X (Steer)"=0.0, "Gyro In Range?"=FALSE, "Distance Drive Finished?"=FALSE, "Stop Eject Lockout"=FALSE, "Dist Drive Status"={"Y In Range"=FALSE, "X In Range"=FALSE, "Gyro In Range"=FALSE, "Y Dist"=0.0, "X Dist"=0.0, "Gyro"=0.0}, "Y Target"=0.0, "Heading Target"=0.0, "Vision Target Aligned?"=FALSE}, "Encoder Values"={"Left Encoder"={"Distance"=0.0, "Speed"=0.0, "Ticks"=0.0}, "Right Encoder"={"Distance"=0.0, "Speed"=0.0, "Ticks"=0.0}}, "IMU Data"={"Pitch"=0.0, "Roll"=0.0, "Yaw"=0.0, "Data Valid?"=FALSE, "Temp"=0.0, "MOVING"=FALSE, "YAW_STABLE"=FALSE, "Accel X"=0.0, "Accel Y"=0.0, "Accel Z"=0.0, "Accel Magnitude"=0.0, "Pitch Rate"=0.0, "Roll Rate"=0.0, "Yaw Rate"=0.0, "NavX Opened?"=FALSE, "Calibration Status"=0, "OP Status"=0}, "Power and Diagnostic Data"={"PDP Data"={"Battery Voltage"=0.0, "Temperature (degrees C)"=0.0, "Internal Battery R (Ohms)"=0.0, "Energy (J)"=0.0, "Power (W)"=0.0, "Total Current (A)"=0.0, "Battery Voltage Fault"=FALSE, "Temperature Fault"=FALSE, "Hardware Fault"=FALSE, "Currents"={"[0]"=0.0, "[1]"=0.0, "[2]"=0.0, "[3]"=0.0, "[4]"=0.0, "[5]"=0.0, "[6]"=0.0, "[7]"=0.0, "[8]"=0.0, "[9]"=0.0, "[10]"=0.0, "[11]"=0.0, "[12]"=0.0, "[13]"=0.0, "[14]"=0.0, "[15]"=0.0}, "Current Faults"={"[0]"=FALSE, "[1]"=FALSE, "[2]"=FALSE, "[3]"=FALSE, "[4]"=FALSE, "[5]"=FALSE, "[6]"=FALSE, "[7]"=FALSE, "[8]"=FALSE, "[9]"=FALSE, "[10]"=FALSE, "[11]"=FALSE, "[12]"=FALSE, "[13]"=FALSE, "[14]"=FALSE, "[15]"=FALSE}}, "PCM Data"={"Compressor Fault"=FALSE, "Solenoid Fault"=FALSE, "Compressor Enabled"=FALSE, "Hardware Fault"=FALSE, "Compressor Current"=0.0}, "roboRIO input voltage (V)"=0.0, "roboRIO input current (A)"=0.0, "3.3V Rail Short"=FALSE, "5 V Rail Short"=FALSE, "6 V Rail Short"=FALSE, "roboRIO Brownout"=FALSE, "Outputs Enabled?"=FALSE}, "Gyro"=0.0, "Intake Status Cluster"={"Roller Power"=0.0, "Angle Power"=0.0, "Intake Mode"=enum."Auto", "Intake States"=enum."Idle", "Rollers Active?"=FALSE, "Current Height"=0.0, "Target Height"=0.0, "Encoder Raw Position"=0.0, "Forward Tripped?"=FALSE, "Backward Tripped?"=FALSE, "Override IR?"=FALSE}, "Ultrasonic Data"={"Left Ultrasonic"=0.0, "Right Ultrasonic"=0.0}, "Climb Status Cluster"={"Pull Power"=0.0, "Unpin Power"=0.0, "PTO Engaged?"=FALSE, "Climb Mode"=enum."Auto"}, "Loop Times"={"DT Loop Timer"=0, "Shooter Loop Timer"=0, "Intake Loop Timer"=0, "US Loop Timer"=0, "Auton File Loop Timer"=0}, "Pressure"=0.0, "Pressure Voltage"=0.0, "Auton Line Number"=0}, binary string=w181) -> (value=w176:T49)  [unwired: 3 in, 2 out]
        n72 = Unbundle By Name(w184) -> ("Robot IP"=→"Robot IP":string, "Camera Addr"=→"Camera IP":string)
        n73 = Unbundle By Name(w176) -> ("Auton Command Cluster"=→"Auton Command Cluster":T7, "Auton File Lists"=→"Auton File Lists":T8, "Encoder Values"=→"Encoder Values":T12, "Drivetrain Status Cluster"=w144:T15, "IMU Data"=w167:T27, "Power and Diagnostic Data"=→"Power and Diagnostic Data":T36, "Gyro"=→"Gyro" →"Gyro 2":dbl, "Intake Status Cluster"=w175:T21, "Climb Status Cluster"=w169:T25, "Loop Times"=→"Loop Times":T43, "Ultrasonic Data"=→"Ultrasonic Data":T29, "Pressure"=→"Pressure":dbl, "Pressure Voltage"=→"Pressure Sensor Voltage":dbl, "Auton Line Number"=→"Line Number":i32)
        "IMU Data" <- w167
        "Intake Status Cluster" <- w175
        "Climb Status Cluster" <- w169
        "Drivetrain Status Cluster" <- w144
        n74 = disable-structure shown="Disabled" {
          disable-tunnel: _ -> [w195 _]
          frame Disabled {
            n75 = Unbundle By Name(w195) -> ("Right RPM"=w188, "Left RPM"=w189, "Angle Ready?"=w194, "RPM Ready?"=w193, "Vision Ready?"=w192, "Ball Loaded?"=w191, "Shooter Ready?"=w190, "State"=w201, "Mode"=w200)
            n76 = case shown="\"Shooter Ready\"" w201 {
              tunnel: ["Idle" "Warmup" "Shooter Ready" "Shooting"] -> w196
              tunnel: [u32 3381759 u32 16746240 u32 16711680 u32 6618880] -> w199
              frame "Idle", Default {
              }
              frame "Warmup" {
              }
              frame "Shooter Ready" {
              }
              frame "Shoot" {
              }
            }
            n77 = case shown="\"Auto\"" w200 {
              tunnel: ["Manual" "Safe" "Auto"] -> w203
              tunnel: [u32 16711680 u32 16770560 u32 6618880] -> w204
              frame "Auto", Default {
              }
              frame "Auto" {
              }
              frame "Auto" {
              }
            }
            n78 = Bundle(w204, w204) -> (w202:cluster{u32, u32})  [unwired: 1 in]
            n79 = Bundle(w199, w199) -> (w198:cluster{u32, u32})  [unwired: 1 in]
            n80 = Build Array(w202) -> ()  [unwired: 1 out]
            n81 = Build Array(w198) -> (w197:cluster{u32, u32}[])
          }
          frame Enabled {
          }
        }
        n82 = Unbundle By Name(w144) -> ("Modes"=w160:T16)
        n83 = Unbundle By Name(w167) -> ("Calibration Status"=→"navX Calibration Status":T5)
        n84 = Unbundle By Name(w175) -> ("Intake States"=w162:T23, "Intake Mode"=w172:T22)
        n85 = case shown="\"Manual\", Default" w160 {
          tunnel: ["Manual" "Climb" "Goal Target" "PID Drive" "Hybrid Drive"] -> w158
          tunnel: [u32 16711680 u32 16770560 u32 6618880 u32 9263615 u32 16743698] -> w159
          frame "Manual", Default {
          }
          frame "Climb" {
          }
          frame "Goal Vision Targeting" {
          }
          frame "PID Distance Drive" {
          }
          frame "Hybrid" {
          }
        }
        n86 = Unbundle By Name(w169) -> ("Climb Mode"=w151:T26)
        n87 = case shown="\"Go Hard or Go Home\"" w162 {
          tunnel: ["Idle" "Rolling Rollers" "Moving to Angle" "Escape Death"] -> w166
          tunnel: [u32 3381759 u32 16746240 u32 16711680 u32 14309887] -> w165
          frame "Idle", Default {
          }
          frame "Set roller speed" {
          }
          frame "Move to angle" {
          }
          frame "Go Hard or Go Home" {
          }
        }
        n88 = case shown="\"Semi-Auto\"" w151 {
          tunnel: ["Manual" "Auto" "Semi-Auto"] -> w155
          tunnel: [u32 16711680 u32 6618880 u32 16770560] -> w152
          frame "Manual", Default {
          }
          frame "Auto" {
          }
          frame "Semi-Auto" {
          }
        }
        n89 = case shown="\"Manual\", Default" w172 {
          tunnel: ["Manual" "Safe" "Auto"] -> w170
          tunnel: [u32 16711680 u32 16770560 u32 6618880] -> w173
          frame "Manual", Default {
          }
          frame "Safe" {
          }
          frame "Auto" {
          }
        }
        n90 = Bundle(w159, w159) -> (w156:cluster{u32, u32})  [unwired: 1 in]
        n91 = Build Array(w156) -> (w157:cluster{u32, u32}[])
        n92 = Bundle(w165, w165) -> (w164:cluster{u32, u32})  [unwired: 1 in]
        n93 = Build Array(w164) -> (w163:cluster{u32, u32}[])
        n94 = Bundle(w152, w152) -> (w153:cluster{u32, u32})  [unwired: 1 in]
        n95 = property on="Drivetrain Mode" class="Bool (strict)"("BoolText.Text"=w158, "Colors [4]"=w157) -> ()  [unwired: 2 in, 2 out]
        n96 = property on="Intake State" class="Bool (strict)"("Colors [4]"=w163, "BoolText.Text"=w166) -> ()  [unwired: 2 in, 2 out]
        n97 = Bundle(w173, w173) -> (w174:cluster{u32, u32})  [unwired: 1 in]
        n98 = Build Array(w153) -> (w154:cluster{u32, u32}[])
        n99 = Build Array(w174) -> (w171:cluster{u32, u32}[])
        n100 = property on="Climb Mode" class="Bool (strict)"("BoolText.Text"=w155, "Colors [4]"=w154) -> ()  [unwired: 2 in, 2 out]
        n101 = property on="Intake Mode" class="Bool (strict)"("BoolText.Text"=w170, "Colors [4]"=w171) -> ()  [unwired: 2 in, 2 out]
        "Control Info" <- w187
        "Status Info" <- w186
        "Robot Metrics" <- w185
        "DS TCP" <- w184
      }
    }
  }
  n102 = while {
    stop <- FALSE stop-if-true
    n103 = Bundle By Name(cluster=T50 {"Encoder Control"={"Right Tick Constant"=0.0, "Left Tick Constant"=0.0, "Reset?"=FALSE, "Y Dist"={"PID gains"={"proportional gain (Kc)"=0.0, "integral time (Ti, min)"=0.0, "derivative time (Td, min)"=0.0}}, "Y Stop Thresh"=0.0, "Y Stop Speed"=0.0}, "Steer PID output"={"output high"=0.0, "output low"=0.0}, " Steer PID gains"={"proportional gain (Kc)"=0.0, "integral time (Ti, min)"=0.0, "derivative time (Td, min)"=0.0}, "Drivetrain Settings"={"Gyro Tolerance"=0.0, "Throttle Ramp (ms)"=0.0, "Kv"=0.0, "Ka"=0.0, "Feed Forward P"=0.0, "Feed Forward D"=0.0, "Goal Vision PID gains"={"proportional gain (Kc)"=1.0, "integral time (Ti, min)"=0.01, "derivative time (Td, min)"=0.0}, "Goal Detection Window"=0.0, "Creep Rate"=0.0, "Vision Throttle Threshold"=0.0, "Min Turn Output"=0.0, "Left Batter Angle"=0.0, "Right Batter Angle"=0.0}, "Vision Packet"={"Distance"=0.0, "Center X"=0.0, "Center Y"=0.0, "Found Target?"=FALSE, "Robot Center"=0.0, "Angle"=0.0}, "Dashboard Drivetrain Command"={"Drivetrain Vision"={"Goal Window"=0.0, "Ball Window"=0.0}}, "Info/Command Cluster"={"Distance to Ball"=0.0, "Desired Angle"=0.0, "Command"=enum."Turn to Ball", "Pixels from Center"=0.0}, "Ball Vision Packet"={"Ball Detected?"=FALSE, "Distance to Ball"=0.0, "Desired Angle"=0.0, "Pixels from Center"=0.0, "Tracking mode"=enum."Turn to Ball"}, "Intake Presets"={"Intake Speed"=0.0, "Outake Speed"=0.0, "Low Height"=0.0, "Half Height"=0.0, "High Idle Height"=0.0, "Angle Speed"=0.0, "Angle Tolerance"=0.0, "Encoder Scale"=0.0, "Load Height"=0.0, "Output Range"={"output high"=0.0, "output low"=0.0}, "Rotation Power Max/Min"=0.0, "MaxCurrent"=0.0, "Intake Trip Time"=0.0, "Idle Height"=0.0, "Max Height"=0.0, "Reset Encoders?"=FALSE, "PID gains"={"proportional gain (Kc)"=0.0, "integral time (Ti, min)"=0.0, "derivative time (Td, min)"=0.0}, "Intake Stop Delay"=0, "Settle Time"=0.0, "Settle Wait Time"=0.0, "Pull Up Delay"=0.0}, "Intake Encoder Control"={"Arm Tick Constant"=0.0, "Reset?"=FALSE, "Y Dist"={"PID gains"={"proportional gain (Kc)"=0.0, "integral time (Ti, min)"=0.0, "derivative time (Td, min)"=0.0}}, "Y Stop Thresh"=0.0, "Y Stop Speed"=0.0}, "Climb Presets"={"Pull Power"=0.0, "Extend Power"=0.0}, "Goal Output Range"={"output high"=0.0, "output low"=0.0}, "Enabled Systems"={"Shoot"=TRUE, "Intake"=TRUE, "DT"=TRUE, "Gyro"=TRUE, "100ms"=TRUE, "US"=TRUE}, "Auton Presets"={"Pitch Limit"=0.0, "Roll Limit"=0.0, "Start Position"=0.0, "Cross Position"=0.0}, "Pressure M"=0.0, "Pressure B"=0.0, "Vision Timeout"=0.0, "Auto-Shift"={"Delay"=0.0, "Speed Thresh"=0.0, "Upshift Accel"=0.0, "Upshift Throttle"=0.0, "Upshift Throttle Accel"=0.0, "Downshift Throttle"=0.0, "Downshift Throttle Accel"=0.0, "Pressure Threshold"=0.0}, "Catapult Setpoints"={"Intake Danger Height"=0.0, "Ball Security Delay "=0.0, "High PSI Minimum"=0.0, "Shot Finish Delay"=0.0, "Low PSI Minimum"=0.0, "Idle Ball Security Wait "=0.0}} ("anything"), "Auto-Shift"="Auto-Shift", "Goal Output Range"="Goal Output Range", "Drivetrain Settings"="Drivetrain Settings", "Steer PID output"="Steer PID output", "Steer PID gains"="Steer PID gains", "Intake Presets"="Intake Presets", "Climb Presets"="Climb Presets", "Encoder Control"="Encoder Settings", "Auton Presets"="Auton Presets", "Pressure M"="Pressure M", "Pressure B"="Pressure B", "Vision Timeout"="Vision Timeout", "Catapult Setpoints"="Catapult Setpoints") -> (w263:T50)
    n104 = Flatten To String(anything=w263) -> (data string=w265:string)  [unwired: 3 in, 2 out]
    n105 = Wait (ms)(milliseconds to wait=u32 250) -> ()  [unwired: 1 out]
    n106 = local read "Robot IP"() -> (w267:string)
    n107 = call "DumbDash Send.vi"("Robot IP"=w267, "data string"=w265) -> ()  [unwired: 10 in]
  }
  n108 = while {
    tunnel: w29 -> [w276]
    shift-right: [w268] -> _
    shift-left: w28 -> [w275]
    tunnel: [w274] -> _
    tunnel: w24 -> [w273]
    tunnel: w23 -> [w272]
    tunnel: w22 -> [_]
    tunnel: w19 -> [w271]
    shift-right: [w269] -> _
    shift-left: _ -> [w270]
    i -> [w274]
    stop <- FALSE stop-if-true
    n109 = event shown="[0] \"Rec Mode\": Value Change" {
      selector: w272 -> [_ _ _]
      dyn-events: [w280 _ _] -> _
      timeout: _ -> [_ _ _]
      tunnel: w276 -> [_ _ _]
      tunnel: w275 -> [w285 _ _]
      tunnel: w273 -> [w284 _ w298]
      tunnel: w271 -> [w283 _ _]
      tunnel: w270 -> [_ _ _]
      tunnel: [0 _ _] -> w269
      tunnel: [w285 _ _] -> w268
      event "Rec Mode": Value Change {
        n110 = event-data() -> ("NewVal"=w278:enum32{"Stop", "Record", "Playback"})  [unwired: 1 in]
        n111 = case shown="\"Playback\"" w278 {
          tunnel: w284 -> [_ w288 w292]
          tunnel: [_ _ w296] -> w280
          tunnel: [_ _ w295] -> _
          tunnel: w283 -> [_ _ w290]
          tunnel: cluster{i32, i32} {-250, 170} -> [_ _ w289]
          tunnel: [_ _ T58 {"Image Size"=TRUE, "Image Type"=TRUE, "Pixel Value"=TRUE, "ROI Information"=TRUE, "Zoom Factor"=FALSE} ("Image Information Shown:All Elements")] -> _
          tunnel: [_ _ TRUE ("Zoom Factor")] -> _
          frame Default {
          }
          frame "Stop", "Record" {
            # "Place Window too"
            n112 = invoke class="VI" method="FP.Close"(reference=w288) -> (reference out=w287:refnum<vi>)  [unwired: 2 in, 2 out]
            n113 = invoke class="VI" method="Abort VI"(reference=w287) -> ()  [unwired: 2 in, 3 out]
          }
          frame "Playback" {
            n114 = call "Open Playback Panel.vi"("Offset"=w289, "DB VI Ref"=w290, "Playback in"=w292) -> ("Playback out"=w291:refnum<vi>)  [unwired: 8 in]
            n115 = register-events(w291) -> (reference out=w296:refnum<event-registration>, error out=w295:errorcluster)  [unwired: 2 in]
          }
        }
        n116 = global write "WPI_DashboardLogging Global.vi" "Logging Filename"(path "") -> ()
        n117 = global write "WPI_DashboardLogging Global.vi" "Recording"(w278) -> ()
        n118 = call <vilib>:"WPI_DashboardNT Log FieldName Cache.vi"("Operation"=enum16{"Lookup/Add", "Index", "Clear"}."Clear") -> ()  [unwired: 8 in, 3 out]
      }
      event Panel Close {
        w297 = enum32{"Stop", "Record", "Playback"}."Stop" ("Rec Mode")
        n119 = event-data() -> ()  [unwired: 1 in, 4 out]
        n120 = local write "Rec Mode"(w297) -> ()
        n121 = global write "WPI_DashboardLogging Global.vi" "Recording"(w297) -> ()
      }
      event Panel Close {
        n122 = event-data() -> ()  [unwired: 1 in, 4 out]
        n123 = invoke class="VI" method="FP.Close"(reference=w298) -> (reference out=w300:refnum<vi>)  [unwired: 2 in, 2 out]
        n124 = invoke class="VI" method="Abort VI"(reference=w300) -> (error out=w299:errorcluster)  [unwired: 2 in, 2 out]
        n125 = invoke class="VI" method="Abort VI"(error in=w299) -> ()  [unwired: 2 in, 3 out]
      }
    }
  }
  n126 = property class="Pnl"(reference=w26) -> ("Panes[]"=w27:refnum<vi>[])  [unwired: 1 in, 2 out]
  n127 = Index Array(array=w27) -> (element=w25:refnum<vi>)  [unwired: 1 in]
  n128 = while {
    tunnel: w25 -> [w302]
    i -> [w305]
    stop <- FALSE stop-if-true
    n129 = Wait (ms)(milliseconds to wait=u32 100) -> ()  [unwired: 1 out]
    n130 = case shown="\"Record\"" "Rec Mode" {
      tunnel: w305 -> [_ _ w320]
      tunnel: [u32 2829099 ("Base Color") u32 11141120 ("Target Color") w309] -> w301
      frame "Stop", Default {
        # "Reset the color, extra updates don't cost much"
      }
      frame "Record" {
      }
      frame "Playback" {
        # "Playback"
        n131 = Quotient & Remainder(x=w320, y=u32 50 ("milliseconds to wait")) -> (x-y*floor(x/y)=w316:u32)  [unwired: 1 out]
        n132 = Divide(x=w316, y=u32 50 ("milliseconds to wait")) -> (x/y=w313:dbl)
        n133 = Multiply(x=6.283185307179586, y=w313) -> (x*y=w318:dbl)
        n134 = Sine(x=w318) -> (sin(x)=w317:dbl)
        n135 = Absolute Value(x=w317) -> (abs(x)=w310:dbl)
        n136 = call "Interpolate RGB Color.vi"("Proportion"=w310, "Target Color"=u32 30976, "Base Color"=u32 2829099) -> ("Result Color"=w309:u32)  [unwired: 8 in]
      }
    }
    n137 = property class="Pane"(reference=w302, "PaneColor"=w301) -> ()  [unwired: 1 in, 2 out]
  }
  n138 = global write "WPI_DashboardLogging Global.vi" "Recording"(w10) -> ()
  n139 = local write "Rec Mode"(w10) -> ()
  n140 = disable-structure shown="Disabled" {
    frame Disabled {
      w323 = T44 4 items=["Grayscale (U8)", "Grayscale (I16)", "Grayscale (SGL)", "Complex (CSG)", "RGB (U32)", "HSL (U32)", "RGB (U64)", "Grayscale (U16)"] ("Image Type")
      n141 = call "IMAQ Create"("Image Name"="Ball Watcher", "Image Type"=w323) -> ("New Image"=w321:T4)  [unwired: 3 in, 1 out]
      n142 = while {
        tunnel: w321 -> [w325]
        stop <- FALSE stop-if-true
        n143 = local read "Camera IP"() -> (w331:string)
        n144 = local read "Rec Mode"() -> (w332:enum32{"Stop", "Record", "Playback"})
        n145 = call "624WPI_CameraRead MJPG for Dashboard.vi"("Camera Settings"="Ball Camera Settings", "Rec Mode"=w332, "Camera IP"=w331, "Camera Mode"="Camera Mode 2", "Refnum in"=w325) -> ("Active"=w333:bool, "Refnum out"=w327:T4, "FPS"=w328:dbl, "Bandwidth (Mbps)"=w329:dbl)  [unwired: 3 in]
        "Ball Cam Active?" <- w333
        n146 = case shown="True" w333 {
          tunnel: w327 -> [_ w335]
          tunnel: w328 -> [_ w337]
          tunnel: w329 -> [_ w336]
          frame False {
            n147 = Wait Until Next ms Multiple(millisecond multiple=u32 500) -> ()  [unwired: 1 out]
          }
          frame True {
            "Front Camera Display 2" <- w335
            "FPS 2" <- w337
            "Bandwidth (Mbps) 2" <- w336
            "Front Camera Display 3" <- w335
          }
        }
      }
    }
    frame Enabled {
    }
  }
  n148 = while {
    tunnel: u16 1741 ("timeout ms (25000)") -> [w339]
    stop <- FALSE stop-if-true
    n149 = TCP Create Listener(10:w339) -> (0:w338:errorcluster, 3:w340:refnum<k5>)  [unwired: 4 in, 1 out]
    n150 = case shown="No Error" w338 {
      selector: w338 -> [w342 _]
      tunnel: w340 -> [w343 _]
      frame No Error {
        n151 = while {
          tunnel: w343 -> [w346]
          tunnel: w342 -> [w345]
          stop <- FALSE stop-if-true
          n152 = TCP Wait On Listener(8:w345, 11:w346) -> (0:w347:errorcluster, 4:w348:refnum<k5>)  [unwired: 2 in, 3 out]
          n153 = local write "TCP"(w348) -> ()
          n154 = case shown="No Error" w347 {
            frame No Error {
            }
            frame Error {
              n155 = Wait (ms)(milliseconds to wait=u32 1000) -> ()  [unwired: 1 out]
            }
          }
        }
      }
      frame Error {
        n156 = Wait (ms)(milliseconds to wait=u32 1000) -> ()  [unwired: 1 out]
      }
    }
  }
  n157 = call <vilib>:"Intialize Keyboard.vi"() -> ("device ID"=w9:refnum<k1>)  [unwired: 10 in, 1 out]
  n158 = while {
    stop <- FALSE stop-if-true
    n159 = local read "IMU Data"() -> (w362:T27)
    n160 = local read "Mode"() -> (w358:T3)
    n161 = Unbundle By Name(w362) -> ("Data Valid?"=w361:bool)
    n162 = Equal?(x=w358, y=T3."Disconnected") -> (x = y?=w355:bool)
    n163 = Equal?(x=w358, y=T3."No Code") -> (x = y?=w356:bool)
    n164 = Or(x=w355, y=w356) -> (x .or. y?=w357:bool)
    n165 = Or(x=w361, y=w357) -> (x .or. y?=w354:bool)
    n166 = case shown="False" w354 {
      tunnel: [w363 u32 2829099 ("Base Color")] -> w351
      frame False {
        n167 = Tick Count (ms)() -> (millisecond timer value=w364:u32)
        n168 = Quotient & Remainder(x=w364, y=u32 1000 ("milliseconds to wait")) -> (x-y*floor(x/y)=w371:u32)  [unwired: 1 out]
        n169 = Divide(x=w371, y=u32 1000 ("milliseconds to wait")) -> (x/y=w368:dbl)
        n170 = Multiply(x=6.283185307179586, y=w368) -> (x*y=w373:dbl)
        n171 = Sine(x=w373) -> (sin(x)=w372:dbl)
        n172 = Absolute Value(x=w372) -> (abs(x)=w367:dbl)
        n173 = call "Interpolate RGB Color.vi"("Proportion"=w367, "Target Color"=u32 16711680, "Base Color"=u32 2829099) -> ("Result Color"=w363:u32)  [unwired: 8 in]
      }
      frame True {
      }
    }
    n174 = property on="Gyro" class="Knob (strict)"("BGColor"=w351) -> ()  [unwired: 2 in, 2 out]
    n175 = property on="Gyro 2" class="Knob (strict)"("BGColor"=w351) -> ()  [unwired: 2 in, 2 out]
    n176 = Wait (ms)(milliseconds to wait=u32 50) -> ()  [unwired: 1 out]
  }
  n177 = while {
    tunnel: w9 -> [w380]
    stop <- FALSE stop-if-true
    n178 = local read "Robot IP"() -> (w378:string)
    n179 = call-poly <vilib>:"Acquire Input Data.vi"("device ID"=w380) -> ("keys pressed"=w379:T59)  [unwired: 16 in, 2 out]
    n180 = call "Send Keyboard Data.vi"("Robot IP"=w378, "keys pressed"=w379) -> ()  [unwired: 10 in]
    n181 = Wait (ms)(milliseconds to wait=50) -> ()  [unwired: 1 out]
  }
  n182 = global write "WPI_DashboardLogging Global.vi" "Recording"(w20) -> ()
  n183 = local write "Rec Mode"(w20) -> ()
  n184 = control-ref of="Dashboard Tab"() -> (w1:refnum<vi>)
  n185 = call "DumbDash Load Controls.vi"("TabControl in"=w1) -> ("Array"=w12:T60[])  [unwired: 10 in]
  n186 = control-ref of="DumbDashMessage"() -> (w11:refnum<vi>)
  n187 = while {
    tunnel: w12 -> [w386]
    tunnel: w11 -> [w384]
    stop <- FALSE stop-if-true
    n188 = disable-structure shown="Enabled" {
      disable-tunnel: ["Robot" Robot_Name."Main Robot" ("Robot")] -> w381
      frame Disabled {
      }
      frame Enabled {
      }
    }
    n189 = Wait (ms)(milliseconds to wait=u32 250) -> ()  [unwired: 1 out]
    n190 = disable-structure shown="RUN_TIME_ENGINE==True" {
      disable-tunnel: "stop" -> [w391 w392]
      frame condition #0 {
        # "Close the build DB"
        n191 = Quit LabVIEW(quit? (T)=w391) -> ()
      }
      frame condition #1 (active) {
        n192 = Stop(stop? (T)=w392) -> ()
      }
    }
    n193 = case shown="True" "Save" {
      tunnel: w386 -> [_ w402]
      tunnel: w384 -> [_ w401]
      tunnel: w381 -> [_ w400]
      frame False {
      }
      frame True {
        n194 = flat-sequence {
          tunnel: w402 -> [w405]
          tunnel: w401 -> [w404]
          tunnel: w400 -> [w403]
          frame #0 {
            n195 = call "DumbDash Save Values.vi"("Message Box"=w404, "Robot"=w403, "Controls In"=w405) -> ()  [unwired: 9 in]
          }
          frame #1 {
            n196 = local write "Save"(FALSE) -> ()
          }
        }
      }
    }
    n197 = case shown="True" "Load" {
      tunnel: w386 -> [_ w395]
      tunnel: w384 -> [_ w394]
      tunnel: w381 -> [_ w393]
      frame False {
      }
      frame True {
        n198 = flat-sequence {
          tunnel: w395 -> [w398]
          tunnel: w394 -> [w397]
          tunnel: w393 -> [w396]
          frame #0 {
            n199 = call "DumbDash Load Values.vi"("Message Box"=w397, "Robot"=w396, "Controls In"=w398) -> ()  [unwired: 9 in]
          }
          frame #1 {
            n200 = local write "Load"(FALSE) -> ()
          }
        }
      }
    }
  }
  n201 = local write "Load"(TRUE) -> ()
